vi "Main.vi"(8 "error in":errorcluster, 11 "TopUI in":refnum<class "TopUI.lvclass">) -> (0 "error out":errorcluster, 3 "TopUI out":refnum<class "TopUI.lvclass">)   [LabVIEW 2019, in "TopUI.lvclass"]
doc: "The <b>Queued Message Handler</b> of the Worker that owns this VI."
uses:
  TopUI.lvclass
  C:/Program Files (x86)/National Instruments/LabVIEW 2019/vi.lib/addons/_Workers/Library/Classes/Worker/Worker.lvclass
  Initialization Data.ctl
  Response Cases.ctl
  rql_AC_Init.ctl
  TopUI.lvclass/TopUI.ctl
  rql_PM_Init.ctl
  rql_Load_Init.ctl
  rql_Rly_Init.ctl
  rql_CK_Type.ctl
  rql_AC_Preset.ctl
  rql_AC_Setup.ctl
  rql_PM_Voltage.ctl
  rql_PM_Current.ctl
  rql_PM_Power.ctl
  rql_PM_P.F.ctl
  rql_PM_Integrate.ctl
  rql_Load_Preset.ctl
  rql_Source_Ctrl.ctl
  rql_Load_Ctrl.ctl
  edbbe92a-6b9d-4f6a-b93a-ee9e5c5b7043.vi
  a3d05794-377f-4d22-b0ed-f270b59c785d.vi
  cac2f185-9852-42f1-bdde-2e867e5f0e86.vi
  326cd913-60c8-4f39-b041-9c4d2d313c5b.vi
  79ea6008-7afc-4004-bcc9-20c1de84bee4.vi
  92421e1f-ff6e-4b36-ba89-2eae84818746.vi
  846e5152-3c31-460c-8b34-4e4e2cc733f6.vi
  63e7fb60-e3b3-40f1-8995-d086ce088de3.vi
  6951fa56-5880-407f-8b78-e7ddc2d94f99.vi
  e5f76952-d3c5-4b56-9ea4-0d04458dc5f7.vi
  <vilib>/Instr/_visa.llb/VISA Configure Serial Port (Instr).vi
  <instrlib>/Yokogawa WT300 Series/Public/Utility/Function/Create Function String (Voltage).vi
  <instrlib>/Yokogawa WT300 Series/Public/Data/Read Measurement (Normal).vi
  <instrlib>/Yokogawa WT300 Series/Public/Utility/Function/Create Function String (Current).vi
  <instrlib>/Yokogawa WT300 Series/Public/Utility/Function/Create Function String (Power).vi
  <instrlib>/Yokogawa WT300 Series/Public/Utility/Function/Create Function String (Integrate).vi
  <vilib>/addons/_Workers/Library/Classes/Message Queue/Message Queue.lvclass
  <instrlib>/Yokogawa WT300 Series/Yokogawa WT300 Series.lvlib
  <instrlib>/Prodigit 331xF Series/Prodigit 331xF Series.lvlib
  <vilib>/addons/_Workers/Debugger/Debug Client/Debug Client.lvlib
panel:
  in  "Load":u16(ring) items=["A,B,C", "D,E,F", "G,H,I"]
  in  "Source":u16(ring) items=["A,B,C", "D,E,F", "G,H,I"]
  in  "InputType":u16(ring) items=["115V,60Hz", "230V,50Hz", "115V,60Hz & 230V,50Hz"]
  in  "OutputType":enum32{"Standard", "TypeC"}(tab)
  in  "MaxLoad":dbl
  in  "Vo":dbl
  in  "Vo_Hi":dbl
  in  "MaxLoad C":dbl
  in  "Initialization Data":T1
  in  "Worker Alias":string="TopUI"
  in  "ST":bool
  in  "Rly":refnum<visa-resource-name>
  in  "Load":refnum<visa-resource-name>
  in  "PM":refnum<visa-resource-name>
  in  "AC":refnum<visa-resource-name>
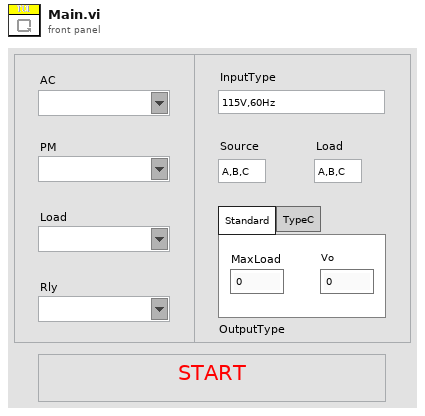
[diagram p1: front panel]
types:
  T1 = typedef "TopUI.lvclass/Initialization Data.ctl" = cluster{"Response Cases":T2}
  T2 = typedef "TopUI.lvclass/Response Cases.ctl" = cluster{"Placeholder - Can be deleted":string}
  T3 = typedef "TopUI.lvclass/rql_AC_Init.ctl" = cluster{"String":string}
  T4 = typedef "TopUI.lvclass/rql_PM_Init.ctl" = cluster{"String":string}
  T5 = typedef "TopUI.lvclass/rql_Load_Init.ctl" = cluster{"String":string}
  T6 = typedef "TopUI.lvclass/rql_Rly_Init.ctl" = cluster{"String":string}
  T7 = typedef "TopUI.lvclass/rql_CK_Type.ctl" = cluster{"String":string}
  T8 = typedef "TopUI.lvclass/rql_AC_Preset.ctl" = cluster{"String":string}
  T9 = enum16{":SOUR:RANG LOW;", ":SOUR:RANG HIGH;", ":SOUR:RANG AUTO;"}
  T10 = typedef "TopUI.lvclass/rql_AC_Setup.ctl" = cluster{"String":string}
  T11 = enum16{"SetRange", "SetVoltage", "SetFreq", "OUTP", "TurnOn"}
  T12 = typedef "TopUI.lvclass/rql_PM_Voltage.ctl" = cluster{"String":string}
  T13 = typedef "TopUI.lvclass/rql_PM_Current.ctl" = cluster{"String":string}
  T14 = typedef "TopUI.lvclass/rql_PM_Power.ctl" = cluster{"String":string}
  T15 = typedef "TopUI.lvclass/rql_PM_P.F.ctl" = cluster{"String":string}
  T16 = typedef "TopUI.lvclass/rql_PM_Integrate.ctl" = cluster{"String":string}
  T17 = typedef "TopUI.lvclass/rql_Load_Preset.ctl" = cluster{"String":string}
  T18 = typedef "TopUI.lvclass/rql_Source_Ctrl.ctl" = cluster{"String":string}
  T19 = typedef "TopUI.lvclass/rql_Load_Ctrl.ctl" = cluster{"String":string}
  T20 = cluster{"RangSelect":enum16{":SOUR:RANG LOW;", ":SOUR:RANG HIGH;", ":SOUR:RANG AUTO;"}, "Volt(V)":string, "Freq(Hz)":string, "OutpSlect":enum16{":SOUR:TURN OFF;", ":SOUR:TURN ON;"}, "TurnSlect":enum16{":SOUR:TURN OFF;", ":SOUR:TURN ON;"}}
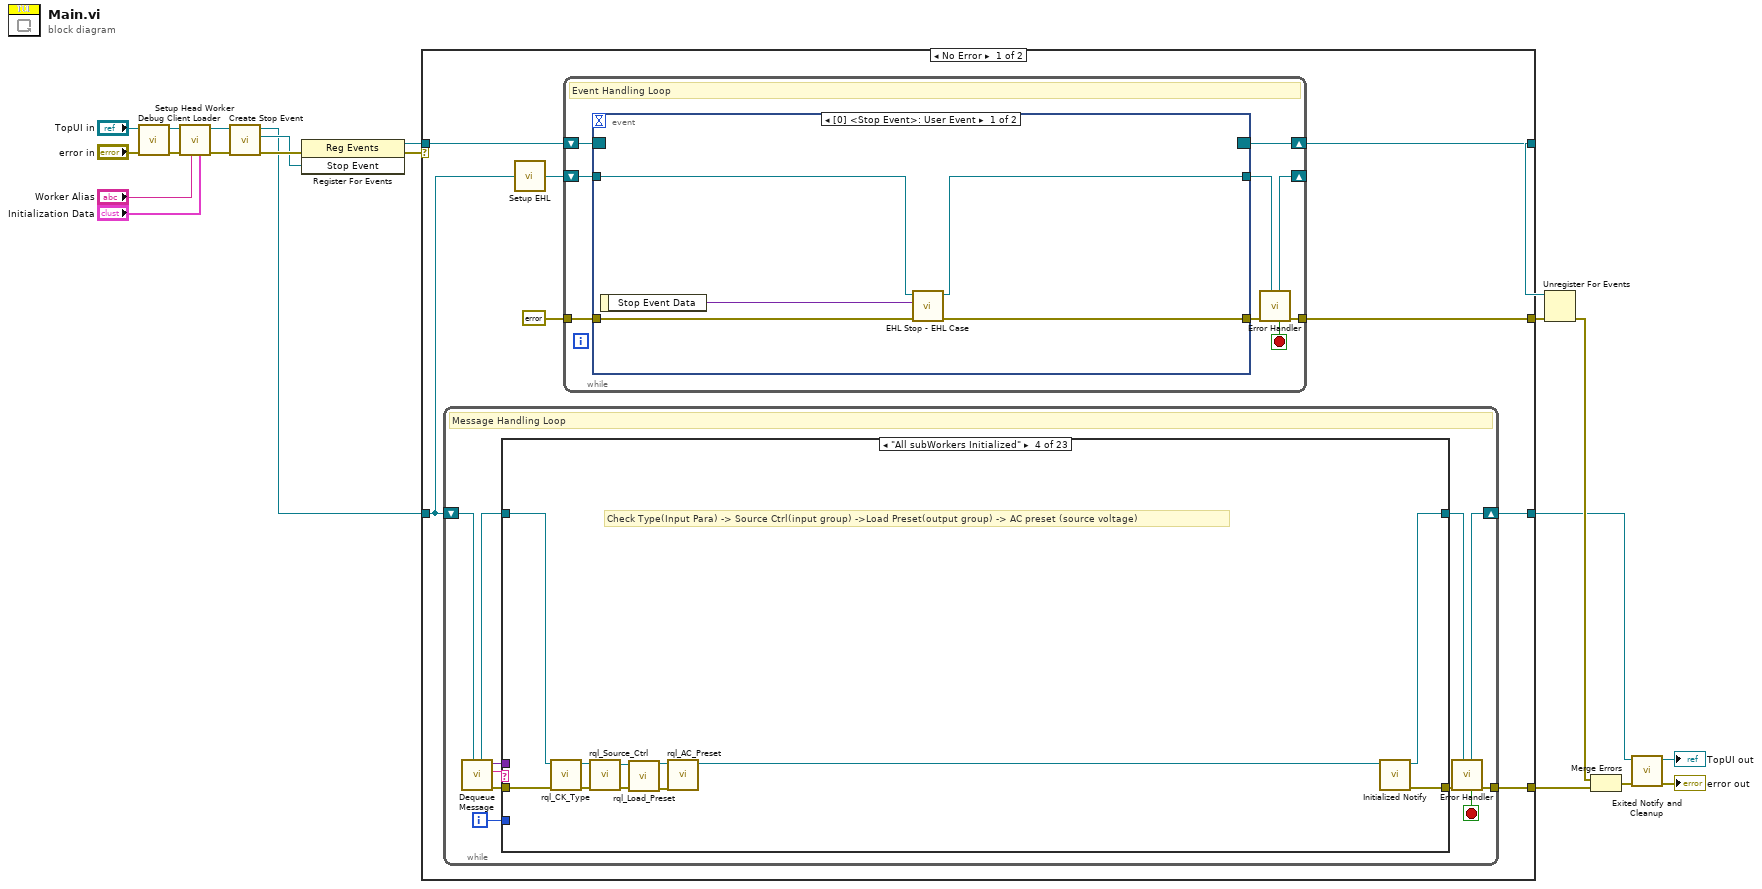
[diagram p0: block diagram]
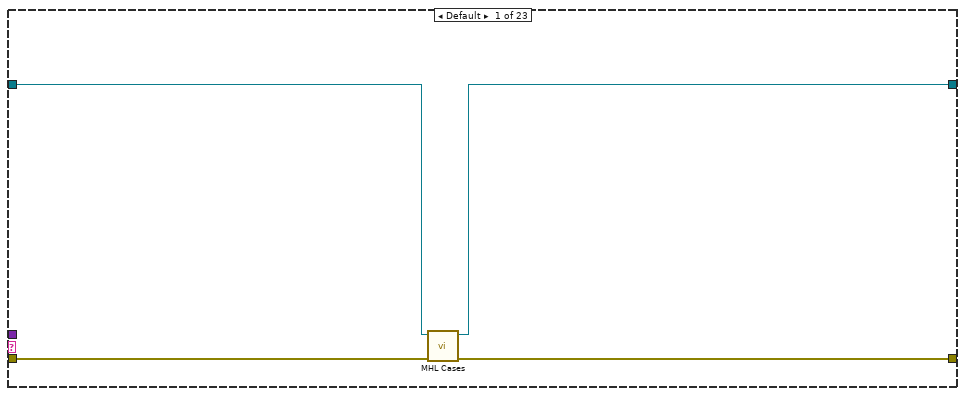
[diagram p2: hidden frame]
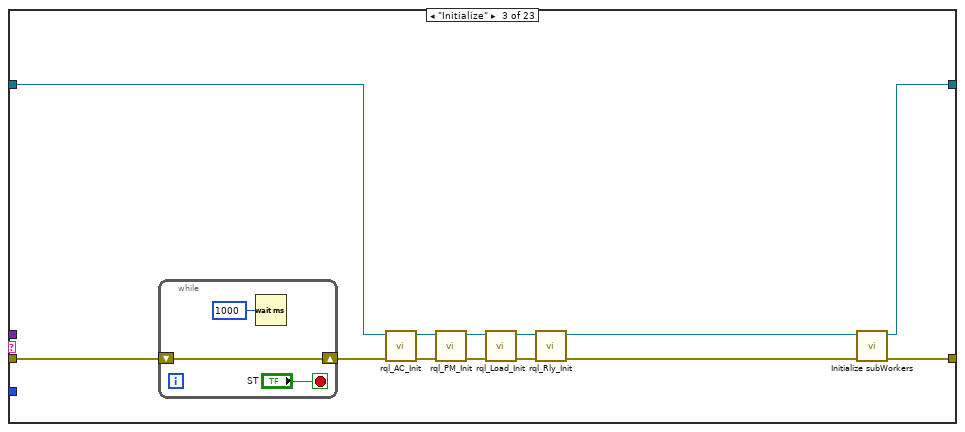
[diagram p4: hidden frame]
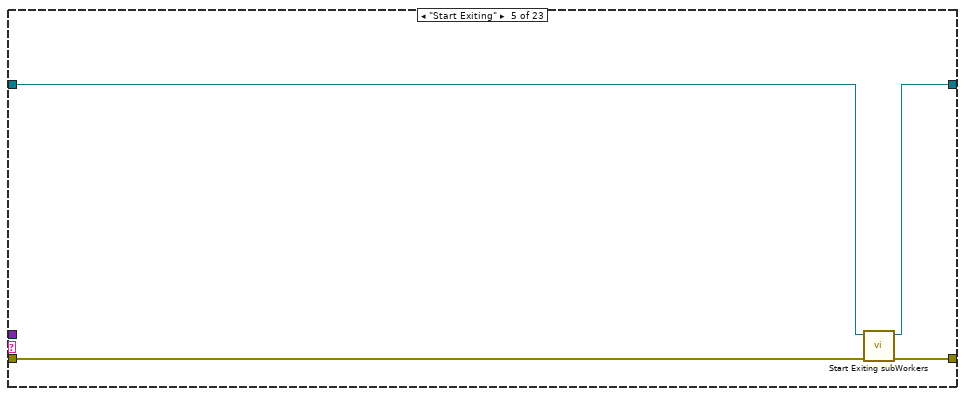
[diagram p5: hidden frame]
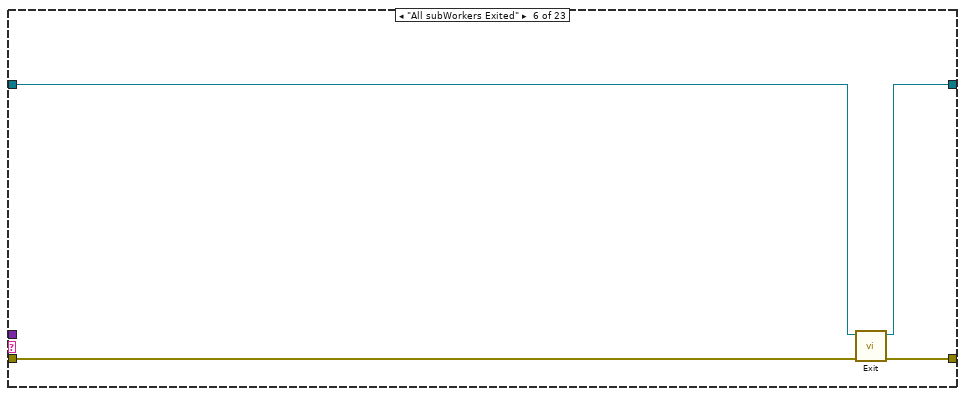
[diagram p6: hidden frame]
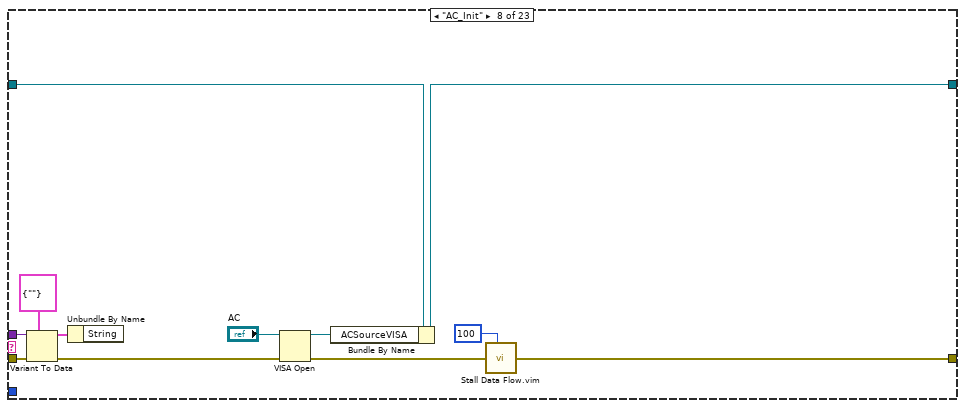
[diagram p8: hidden frame]
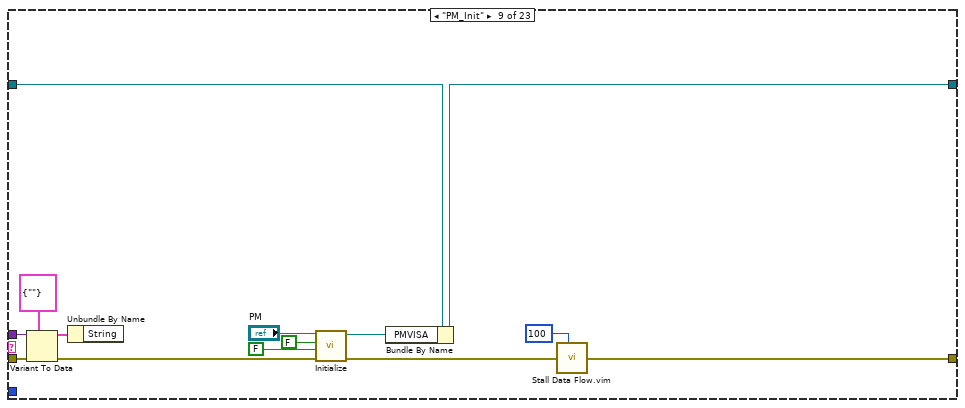
[diagram p9: hidden frame]
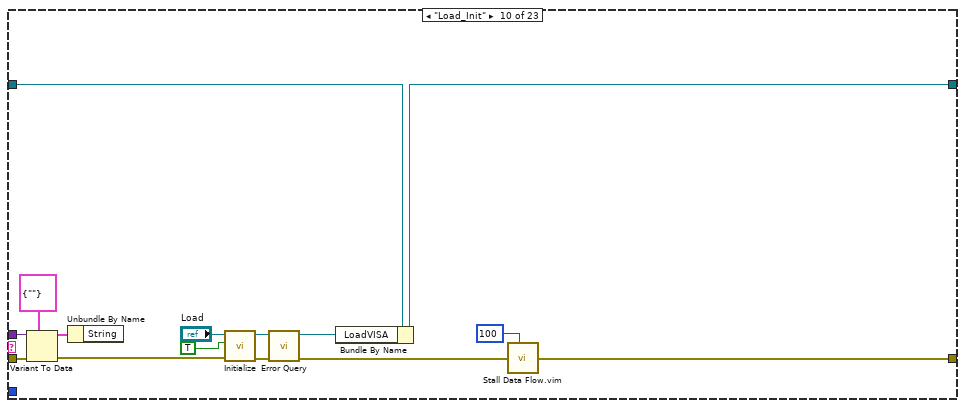
[diagram p10: hidden frame]
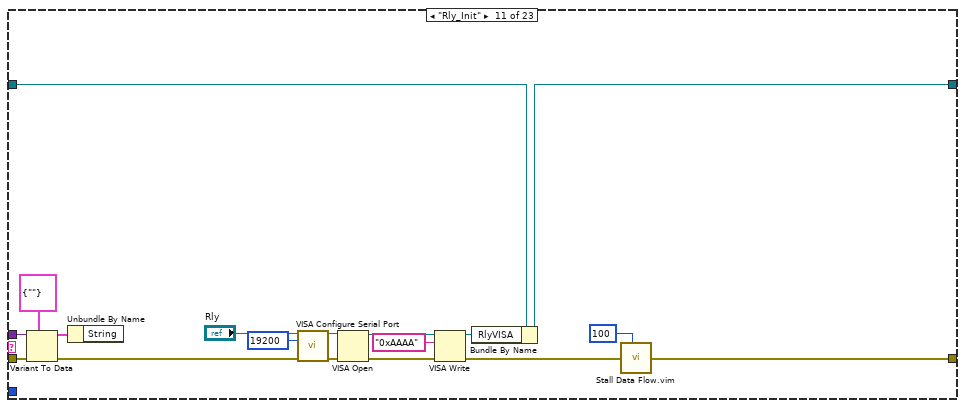
[diagram p11: hidden frame]
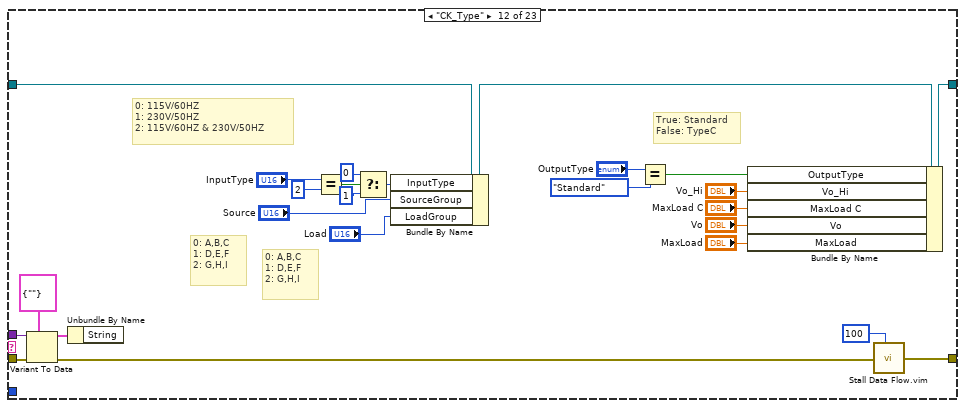
[diagram p12: hidden frame]
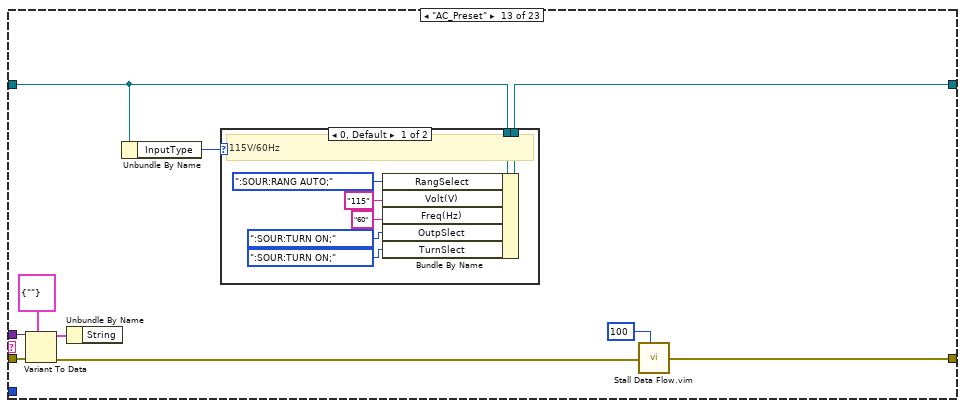
[diagram p13: hidden frame]
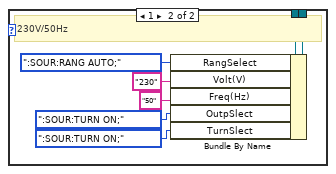
[diagram p14: hidden frame]
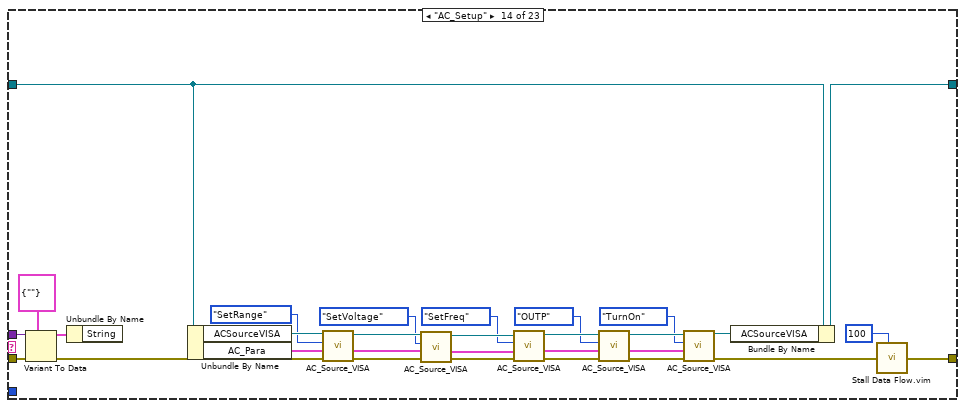
[diagram p15: hidden frame]
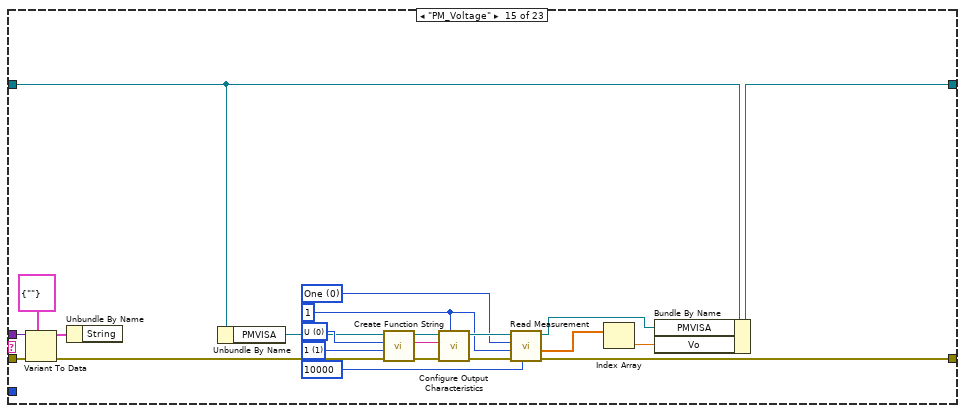
[diagram p16: hidden frame]
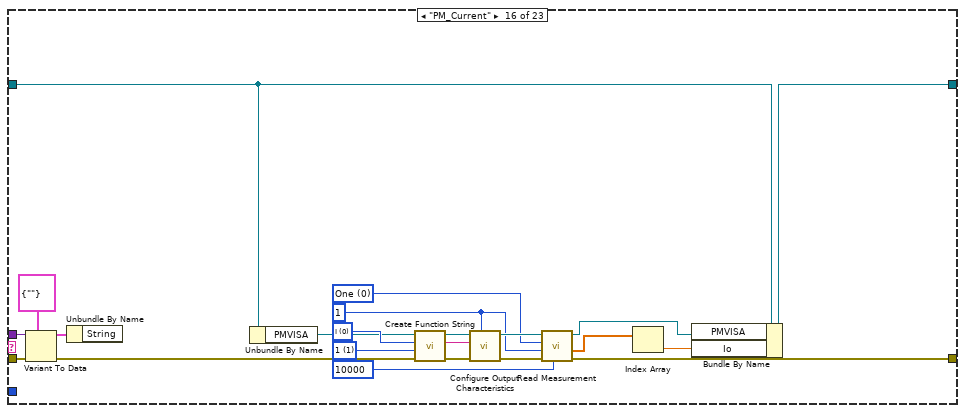
[diagram p17: hidden frame]
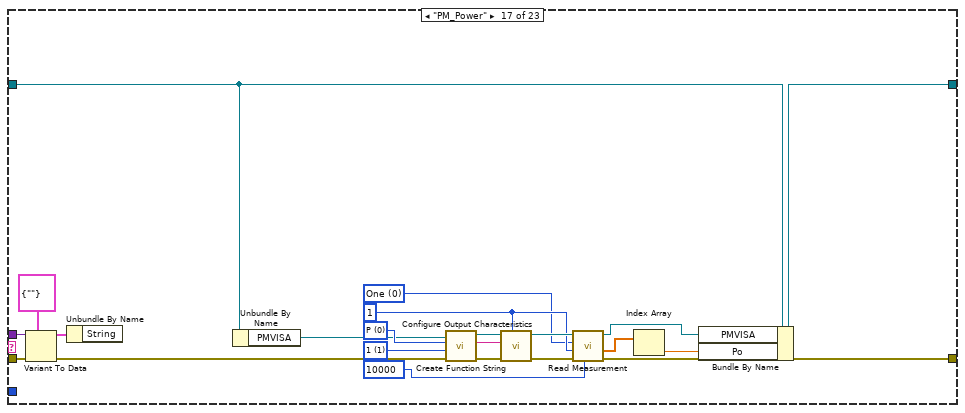
[diagram p18: hidden frame]
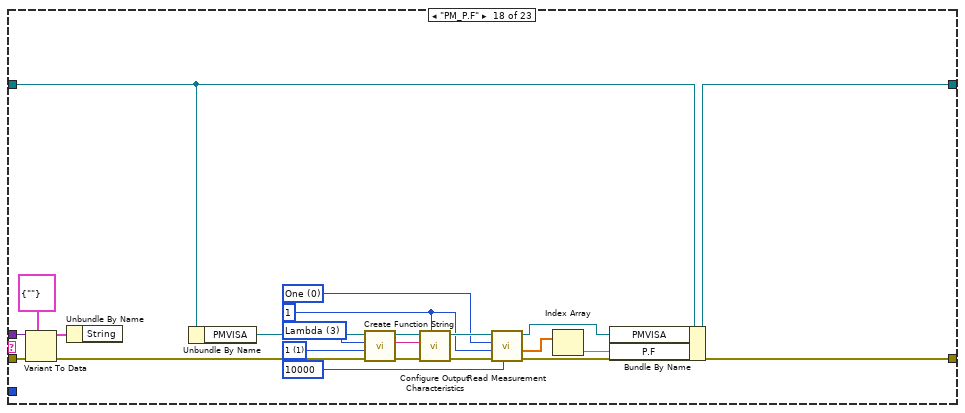
[diagram p19: hidden frame]
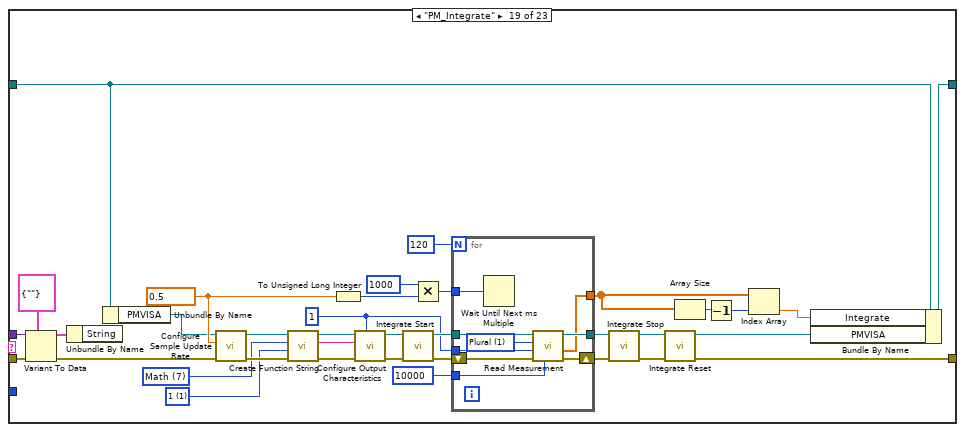
[diagram p20: hidden frame]
diagram:
  n1 = call <vilib>:"Debug Client Loader.vi"("error in (no error)"="error in", "Worker_"="TopUI in") -> ("error out"=w8:errorcluster, "Worker_out"=w7:refnum<class "TopUI.lvclass">)  [unwired: 8 in]
  n2 = call-dynamic "Setup Head Worker.vi"("Initalization Data"="Initialization Data", "Worker Alias"="Worker Alias", "error in"=w8, "Worker_"=w7) -> ("error out"=w3:errorcluster, "Worker_out"=w4:refnum<class "TopUI.lvclass">)  [unwired: 6 in]
  n3 = call-dynamic "Create Stop Event.vi"("error in"=w3, "Worker"=w4) -> ("error out"=w16:errorcluster, "Stop Event"=w13:refnum<user-event>, "Worker out"=w10:refnum<class "TopUI.lvclass">)  [unwired: 7 in]
  n4 = register-events(error in=w16, w13) -> (reference out=w15:refnum<event-registration>, error out=w9:errorcluster)  [unwired: 1 in]
  n5 = case shown="No Error" w9 {
    tunnel: w10 -> [w24 w447]
    tunnel: [w22 w448] -> w14
    tunnel: w15 -> [w29 w449]
    tunnel: [w26 w450] -> w20
    tunnel: [w28 w449] -> w19
    tunnel: [w23 w446] -> w17
    selector: w9 -> [_ w450]
    frame No Error {
      n6 = while {
        shift-right: [w38] -> w23
        shift-left: w24 -> [w40]
        tunnel: [w39] -> w22
        i -> [w31]
        stop <- w32 stop-if-true
        # "Message Handling Loop"
        n7 = call-dynamic "Dequeue Message.vi"("Worker"=w40) -> ("error out"=w37:errorcluster, "Case out"=w33:string, "Data out"=w30:variant, "Worker out"=w35:refnum<class "TopUI.lvclass">)  [unwired: 6 in, 1 out]
        n8 = case "Worker MHL Case Structure (DO NOT CHANGE LABEL NAME)" shown="\"All subWorkers Initialized\"" w33 {
          tunnel: w37 -> [w44 w45 w47 w71 w74 w81 w83 w87 w99 w113 w128 w146 w171 w195 w225 w247 w269 w291 w313 w369 w408 w422 w424]
          tunnel: [w41 w45 w59 w73 w77 w80 w83 w89 w108 w123 w137 w166 w176 w220 w233 w255 w276 w298 w319 w363 w403 w412 w424] -> w36
          tunnel: w35 -> [w43 w46 w49 w70 w75 w79 w82 w92 w104 w117 w136 w159 w174 w199 w230 w252 w274 w296 w324 w362 w402 w410 w423]
          tunnel: [w42 w46 w56 w72 w76 w78 w82 w90 w103 w115 w135 w160 w173 w197 w227 w249 w273 w295 w323 w360 w401 w409 w423] -> w34
          tunnel: w31 -> [_ _ _ _ _ _ _ _ _ _ _ _ _ _ _ _ _ _ _ _ _ _ _]
          tunnel: w30 -> [_ _ _ _ _ _ _ w85 w97 w111 w126 w143 w168 w193 w223 w244 w267 w289 w311 w367 w406 w420 _]
          frame Default {
            # "Base Class MHL Cases\nContains the MHL Cases of this Worker's base class."
            n9 = call-dynamic "MHL Cases.vi"("error in"=w44, "Worker in"=w43) -> ("error out"=w41:errorcluster, "Worker out"=w42:refnum<class "TopUI.lvclass">)  [unwired: 8 in]
          }
          frame "------------ FRAMEWORK CASES -----------" {
            # "Start of Workers Framework Cases"
          }
          frame "Initialize" {
            # "The first user case called when this Worker is loaded.\nThe end of this case (or series of cases) should call 'Initialize subWorkers.vi'"
            n10 = while {
              shift-right: [w62] -> w48
              shift-left: w47 -> [w62]
              stop <- "ST" stop-if-true
              n11 = Wait (ms)(milliseconds to wait=u32 1000) -> ()  [unwired: 1 out]
            }
            n12 = call "rql_AC_Init.vi"("error in"=w48, "TopUI in"=w49) -> ("error out"=w58:errorcluster, "dup TopUI out"=w57:refnum<class "TopUI.lvclass">)  [unwired: 8 in]
            n13 = call "rql_PM_Init.vi"("error in"=w58, "TopUI in"=w57) -> ("error out"=w55:errorcluster, "dup TopUI out"=w54:refnum<class "TopUI.lvclass">)  [unwired: 8 in]
            n14 = call "rql_Load_Init.vi"("error in"=w55, "TopUI in"=w54) -> ("error out"=w53:errorcluster, "dup TopUI out"=w52:refnum<class "TopUI.lvclass">)  [unwired: 8 in]
            n15 = call "rql_Rly_Init.vi"("error in"=w53, "TopUI in"=w52) -> ("error out"=w50:errorcluster, "dup TopUI out"=w51:refnum<class "TopUI.lvclass">)  [unwired: 8 in]
            n16 = call-dynamic "Initialize subWorkers.vi"("error in"=w50, "Worker"=w51) -> ("error out"=w59:errorcluster, "dup Worker out"=w56:refnum<class "TopUI.lvclass">)  [unwired: 8 in]
          }
          frame "All subWorkers Initialized" {
            # "Check Type(Input Para) -> Source Ctrl(input group) ->Load Preset(output group) -> AC preset (source voltage)"
            # "All of this Worker's statically-linked subWorkers have been successfully initialized.\nThis case should now call 'Initialized Notify.vi'"
            n17 = call "rql_CK_Type.vi"("error in"=w71, "TopUI in"=w70) -> ("error out"=w69:errorcluster, "dup TopUI out"=w68:refnum<class "TopUI.lvclass">)  [unwired: 8 in]
            n18 = call "rql_Source_Ctrl.vi"("error in"=w69, "TopUI in"=w68) -> ("error out"=w65:errorcluster, "dup TopUI out"=w66:refnum<class "TopUI.lvclass">)  [unwired: 8 in]
            n19 = call "rql_Load_Preset.vi"("error in"=w65, "TopUI in"=w66) -> ("error out"=w64:errorcluster, "dup TopUI out"=w63:refnum<class "TopUI.lvclass">)  [unwired: 8 in]
            n20 = call "rql_AC_Preset.vi"("error in"=w64, "TopUI in"=w63) -> ("dup TopUI out"=w67:refnum<class "TopUI.lvclass">)  [unwired: 8 in, 1 out]
            n21 = call-dynamic "Initialized Notify.vi"("Worker"=w67) -> ("error out"=w73:errorcluster, "dup Worker out"=w72:refnum<class "TopUI.lvclass">)  [unwired: 9 in]
          }
          frame "Start Exiting" {
            # "This Worker has been requested to exit. \nThe end of this case (or series of cases) should call 'Start Exiting subWorkers.vi'"
            n22 = call-dynamic "Start Exiting subWorkers.vi"("error_in"=w74, "Worker"=w75) -> ("error out"=w77:errorcluster, "dup Worker out"=w76:refnum<class "TopUI.lvclass">)  [unwired: 8 in]
          }
          frame "All subWorkers Exited" {
            # "All of this Worker's subWorkers have successfully exited. \nThe end of this case (or series of cases) should call 'Exit.vi'"
            n23 = call-dynamic "Exit.vi"("error_in"=w81, "Worker"=w79) -> ("error out"=w80:errorcluster, "dup Worker out"=w78:refnum<class "TopUI.lvclass">)  [unwired: 8 in]
          }
          frame "------------- LOCAL API CASES -------------" {
            # "Start of Workers Local API Cases"
          }
          frame "AC_Init" {
            # "Workers Local API Request Case"
            n24 = Variant To Data(error in=w87, type=T3 {"String"=""} ("Data"), Variant=w85) -> (data=w88:T3, error out=w86:errorcluster)
            n25 = Unbundle By Name(w88) -> ()  [unwired: 1 out]
            n26 = VISA Open(error in (no error)=w86, VISA resource name="AC") -> (VISA resource name=w91:refnum<visa-resource-name>, error out=w94:errorcluster)  [unwired: 3 in]
            n27 = Bundle By Name(cluster=w92, "ACSourceVISA"=w91) -> (w90:refnum<class "TopUI.lvclass">)
            n28 = call "Stall Data Flow.vim"("value in"=w94, "milliseconds to wait"=u32 100) -> ("value out"=w89:errorcluster)  [unwired: 1 out]
          }
          frame "PM_Init" {
            # "Workers Local API Request Case"
            n29 = Variant To Data(error in=w99, type=T4 {"String"=""} ("Data"), Variant=w97) -> (data=w100:T4, error out=w96:errorcluster)
            n30 = Unbundle By Name(w100) -> ()  [unwired: 1 out]
            n31 = call <instrlib>:"Initialize.vi"("error in (no error)"=w96, "Reset (True)"=FALSE, "ID Query (True)"=FALSE, "VISA resource name"="PM") -> ("error out"=w105:errorcluster, "VISA resource name out"=w102:refnum<visa-resource-name>)  [unwired: 6 in]
            n32 = Bundle By Name(cluster=w104, "PMVISA"=w102) -> (w103:refnum<class "TopUI.lvclass">)
            n33 = call "Stall Data Flow.vim"("value in"=w105, "milliseconds to wait"=u32 100) -> ("value out"=w108:errorcluster)  [unwired: 1 out]
          }
          frame "Load_Init" {
            # "Workers Local API Request Case"
            n34 = Variant To Data(error in=w113, type=T5 {"String"=""} ("Data"), Variant=w111) -> (data=w114:T5, error out=w112:errorcluster)
            n35 = Unbundle By Name(w114) -> ()  [unwired: 1 out]
            n36 = call <instrlib>:"Initialize.vi"("error in (no error)"=w112, "ID Query (True)"=TRUE, "VISA resource name"="Load") -> ("error out"=w119:errorcluster, "VISA resource name out"=w122:refnum<visa-resource-name>)  [unwired: 7 in]
            n37 = call <instrlib>:"Error Query.vi"("error in (no error)"=w119, "VISA resource name"=w122) -> ("error out"=w118:errorcluster, "VISA resource name out"=w116:refnum<visa-resource-name>)  [unwired: 6 in, 2 out]
            n38 = Bundle By Name(cluster=w117, "LoadVISA"=w116) -> (w115:refnum<class "TopUI.lvclass">)
            n39 = call "Stall Data Flow.vim"("value in"=w118, "milliseconds to wait"=u32 100) -> ("value out"=w123:errorcluster)  [unwired: 1 out]
          }
          frame "Rly_Init" {
            # "Workers Local API Request Case"
            n40 = Variant To Data(error in=w128, type=T6 {"String"=""} ("Data"), Variant=w126) -> (data=w129:T6, error out=w127:errorcluster)
            n41 = Unbundle By Name(w129) -> ()  [unwired: 1 out]
            n42 = call-poly "VISA Configure Serial Port"("VISA resource name"="Rly", "baud rate (9600)"=u32 19200, "error in (no error)"=w127) -> ("VISA resource name out"=w141:refnum<visa-resource-name>, "error out"=w142:errorcluster)  [unwired: 6 in, 5 out]
            n43 = VISA Open(error in (no error)=w142, VISA resource name=w141) -> (VISA resource name=w131:refnum<visa-resource-name>, error out=w134:errorcluster)  [unwired: 3 in]
            n44 = VISA Write(VISA resource name=w131, write buffer="0xAAAA", error in (no error)=w134) -> (VISA resource name out=w132:refnum<visa-resource-name>, error out=w133:errorcluster)  [unwired: 1 out]
            n45 = Bundle By Name(cluster=w136, "RlyVISA"=w132) -> (w135:refnum<class "TopUI.lvclass">)
            n46 = call "Stall Data Flow.vim"("value in"=w133, "milliseconds to wait"=u32 100) -> ("value out"=w137:errorcluster)  [unwired: 1 out]
          }
          frame "CK_Type" {
            # "0: A,B,C\n1: D,E,F\n2: G,H,I"
            # "0: A,B,C\n1: D,E,F\n2: G,H,I"
            # "True: Standard\nFalse: TypeC"
            # "0: 115V/60HZ\n1: 230V/50HZ\n2: 115V/60HZ & 230V/50HZ"
            # "Workers Local API Request Case"
            n47 = Variant To Data(error in=w146, type=T7 {"String"=""} ("Data"), Variant=w143) -> (data=w147:T7, error out=w145:errorcluster)
            n48 = Unbundle By Name(w147) -> ()  [unwired: 1 out]
            n49 = Equal?(x="InputType", y=u16 2) -> (x = y?=w155:bool)
            n50 = Select(t=u16 0 ("y"), s=w155, f=u16 1 ("y")) -> (s? t:f=w152:u16)
            n51 = Bundle By Name(cluster=w159, "InputType"=w152, "SourceGroup"="Source", "LoadGroup"="Load") -> (w158:refnum<class "TopUI.lvclass">)
            n52 = Equal?(x="OutputType", y=enum32{"Standard", "TypeC"}."Standard") -> (x = y?=w165:bool)
            n53 = Bundle By Name(cluster=w158, "OutputType"=w165, "Vo_Hi"="Vo_Hi", "MaxLoad C"="MaxLoad C", "Vo"="Vo", "MaxLoad"="MaxLoad") -> (w160:refnum<class "TopUI.lvclass">)
            n54 = call "Stall Data Flow.vim"("value in"=w145, "milliseconds to wait"=u32 100) -> ("value out"=w166:errorcluster)  [unwired: 1 out]
          }
          frame "AC_Preset" {
            # "Workers Local API Request Case"
            n55 = Variant To Data(error in=w171, type=T8 {"String"=""} ("Data"), Variant=w168) -> (data=w172:T8, error out=w170:errorcluster)
            n56 = Unbundle By Name(w172) -> ()  [unwired: 1 out]
            n57 = Unbundle By Name(w174) -> ("InputType"=w175:u16)
            n58 = case shown="0, Default" w175 {
              tunnel: w174 -> [w184 w191]
              tunnel: [w183 w190] -> w173
              frame 0, Default {
                # "115V/60Hz"
                n59 = Bundle By Name(cluster=w184, "RangSelect"=T9.":SOUR:RANG AUTO;" ("AC_Para.RangSelect"), "Volt(V)"="115" ("AC_Para.Volt(V)"), "Freq(Hz)"="60" ("AC_Para.Freq(Hz)"), "OutpSlect"=enum16{":SOUR:TURN OFF;", ":SOUR:TURN ON;"}.":SOUR:TURN ON;" ("AC_Para.OutpSlect"), "TurnSlect"=enum16{":SOUR:TURN OFF;", ":SOUR:TURN ON;"}.":SOUR:TURN ON;" ("AC_Para.TurnSlect")) -> (w183:refnum<class "TopUI.lvclass">)
              }
              frame 1 {
                # "230V/50Hz"
                n60 = Bundle By Name(cluster=w191, "RangSelect"=T9.":SOUR:RANG AUTO;" ("AC_Para.RangSelect"), "Volt(V)"="230" ("AC_Para.Volt(V)"), "Freq(Hz)"="50" ("AC_Para.Freq(Hz)"), "OutpSlect"=enum16{":SOUR:TURN OFF;", ":SOUR:TURN ON;"}.":SOUR:TURN ON;" ("AC_Para.OutpSlect"), "TurnSlect"=enum16{":SOUR:TURN OFF;", ":SOUR:TURN ON;"}.":SOUR:TURN ON;" ("AC_Para.TurnSlect")) -> (w190:refnum<class "TopUI.lvclass">)
              }
            }
            n61 = call "Stall Data Flow.vim"("value in"=w170, "milliseconds to wait"=u32 100) -> ("value out"=w176:errorcluster)  [unwired: 1 out]
          }
          frame "AC_Setup" {
            # "Workers Local API Request Case"
            n62 = Variant To Data(error in=w195, type=T10 {"String"=""} ("Data"), Variant=w193) -> (data=w196:T10, error out=w194:errorcluster)
            n63 = Unbundle By Name(w196) -> ()  [unwired: 1 out]
            n64 = Unbundle By Name(w199) -> ("ACSourceVISA"=w219:refnum<visa-resource-name>, "AC_Para"=w218:T20)
            n65 = call "AC_Source_VISA.vi"("error_in"=w194, "Parameter"=w218, "Mode"=T11."SetRange", "VISA_in"=w219) -> ("error_out"=w216:errorcluster, "Parameter 2"=w208:T20, "VISA_out"=w215:refnum<visa-resource-name>)  [unwired: 1 in]
            n66 = call "AC_Source_VISA.vi"("error_in"=w216, "Parameter"=w208, "Mode"=T11."SetVoltage", "VISA_in"=w215) -> ("error_out"=w213:errorcluster, "Parameter 2"=w207:T20, "VISA_out"=w214:refnum<visa-resource-name>)  [unwired: 1 in]
            n67 = call "AC_Source_VISA.vi"("error_in"=w213, "Parameter"=w207, "Mode"=T11."SetFreq", "VISA_in"=w214) -> ("error_out"=w211:errorcluster, "Parameter 2"=w206:T20, "VISA_out"=w212:refnum<visa-resource-name>)  [unwired: 1 in]
            n68 = call "AC_Source_VISA.vi"("error_in"=w211, "Parameter"=w206, "Mode"=T11."OUTP", "VISA_in"=w212) -> ("error_out"=w209:errorcluster, "Parameter 2"=w205:T20, "VISA_out"=w210:refnum<visa-resource-name>)  [unwired: 1 in]
            n69 = call "AC_Source_VISA.vi"("error_in"=w209, "Parameter"=w205, "Mode"=T11."TurnOn", "VISA_in"=w210) -> ("error_out"=w204:errorcluster, "VISA_out"=w198:refnum<visa-resource-name>)  [unwired: 1 in, 1 out]
            n70 = Bundle By Name(cluster=w199, "ACSourceVISA"=w198) -> (w197:refnum<class "TopUI.lvclass">)
            n71 = call "Stall Data Flow.vim"("value in"=w204, "milliseconds to wait"=u32 100) -> ("value out"=w220:errorcluster)  [unwired: 1 out]
          }
          frame "PM_Voltage" {
            w235 = 1 items=["1"=1, "2"=2, "3"=3, "Sigma A"=4] ("Element (1: 1)")
            w234 = 0 items=["U", "UPPeak", "UMPeak"] ("Function (0: U)")
            w237 = 1 ("Item (1)")
            w236 = 0 items=["One", "Plural"] ("Measure Item")
            # "Workers Local API Request Case"
            n72 = Variant To Data(error in=w225, type=T12 {"String"=""} ("Data"), Variant=w223) -> (data=w226:T12, error out=w224:errorcluster)
            n73 = Unbundle By Name(w226) -> ()  [unwired: 1 out]
            n74 = Unbundle By Name(w230) -> ("PMVISA"=w232:refnum<visa-resource-name>)
            n75 = call-poly <instrlib>:"Create Function String.vi"("error in (no error)"=w224, "Element (1: 1)"=w235, "Function (0: U)"=w234, "VISA resource name"=w232) -> ("error out"=w242:errorcluster, "Function String"=w243:string, "VISA resource name out"=w241:refnum<visa-resource-name>)  [unwired: 5 in]
            n76 = call <instrlib>:"Configure Output Characteristics.vi"("Item (1)"=w237, "error in (no error)"=w242, "Function (Empty)"=w243, "VISA resource name"=w241) -> ("error out"=w240:errorcluster, "VISA resource name out"=w239:refnum<visa-resource-name>)  [unwired: 6 in]
            n77 = call-poly <instrlib>:"Read Measurement.vi"("Timeout (10000 ms)"=10000, "error in (no error)"=w240, "Number of Item (15)"=w237, "Measure Item (1: Plural)"=w236, "VISA resource name"=w239) -> ("error out"=w233:errorcluster, "Measurement"=w231:dbl[], "VISA resource name out"=w229:refnum<visa-resource-name>)  [unwired: 3 in, 1 out]
            n78 = Index Array(array=w231) -> (element=w228:dbl)  [unwired: 1 in]
            n79 = Bundle By Name(cluster=w230, "PMVISA"=w229, "Vo"=w228) -> (w227:refnum<class "TopUI.lvclass">)
          }
          frame "PM_Current" {
            w256 = 0 items=["I", "IPPeak", "IMPeak"] ("Function (0: I)")
            w257 = 1 items=["1"=1, "2"=2, "3"=3, "Sigma A"=4] ("Element (1: 1)")
            w259 = 1 ("Item (1)")
            w258 = 0 items=["One", "Plural"] ("Measure Item")
            # "Workers Local API Request Case"
            n80 = Variant To Data(error in=w247, type=T13 {"String"=""} ("Data"), Variant=w244) -> (data=w248:T13, error out=w246:errorcluster)
            n81 = Unbundle By Name(w248) -> ()  [unwired: 1 out]
            n82 = Unbundle By Name(w252) -> ("PMVISA"=w253:refnum<visa-resource-name>)
            n83 = call-poly <instrlib>:"Create Function String.vi"("error in (no error)"=w246, "Element (1: 1)"=w257, "Function (0: I)"=w256, "VISA resource name"=w253) -> ("error out"=w264:errorcluster, "Function String"=w265:string, "VISA resource name out"=w263:refnum<visa-resource-name>)  [unwired: 5 in]
            n84 = call <instrlib>:"Configure Output Characteristics.vi"("Item (1)"=w259, "error in (no error)"=w264, "Function (Empty)"=w265, "VISA resource name"=w263) -> ("error out"=w262:errorcluster, "VISA resource name out"=w261:refnum<visa-resource-name>)  [unwired: 6 in]
            n85 = call-poly <instrlib>:"Read Measurement.vi"("Timeout (10000 ms)"=10000, "error in (no error)"=w262, "Number of Item (15)"=w259, "Measure Item (1: Plural)"=w258, "VISA resource name"=w261) -> ("error out"=w255:errorcluster, "Measurement"=w254:dbl[], "VISA resource name out"=w251:refnum<visa-resource-name>)  [unwired: 3 in, 1 out]
            n86 = Index Array(array=w254) -> (element=w250:dbl)  [unwired: 1 in]
            n87 = Bundle By Name(cluster=w252, "PMVISA"=w251, "Io"=w250) -> (w249:refnum<class "TopUI.lvclass">)
          }
          frame "PM_Power" {
            w279 = 0 items=["P", "S", "Q", "Lambda", "Phi", "P+peak", "P-peak"] ("Function (0: P)")
            w280 = 1 items=["1"=1, "2"=2, "3"=3, "Sigma A"=4] ("Element (1: 1)")
            w281 = 1 ("Item (1)")
            w277 = 0 items=["One", "Plural"] ("Measure Item")
            # "Workers Local API Request Case"
            n88 = Variant To Data(error in=w269, type=T14 {"String"=""} ("Data"), Variant=w267) -> (data=w270:T14, error out=w268:errorcluster)
            n89 = Unbundle By Name(w270) -> ()  [unwired: 1 out]
            n90 = Unbundle By Name(w274) -> ("PMVISA"=w275:refnum<visa-resource-name>)
            n91 = call-poly <instrlib>:"Create Function String.vi"("error in (no error)"=w268, "Element (1: 1)"=w280, "Function (0: P)"=w279, "VISA resource name"=w275) -> ("error out"=w284:errorcluster, "Function String"=w283:string, "VISA resource name out"=w285:refnum<visa-resource-name>)  [unwired: 5 in]
            n92 = call <instrlib>:"Configure Output Characteristics.vi"("Item (1)"=w281, "error in (no error)"=w284, "Function (Empty)"=w283, "VISA resource name"=w285) -> ("error out"=w286:errorcluster, "VISA resource name out"=w287:refnum<visa-resource-name>)  [unwired: 6 in]
            n93 = call-poly <instrlib>:"Read Measurement.vi"("Timeout (10000 ms)"=10000, "error in (no error)"=w286, "Number of Item (15)"=w281, "Measure Item (1: Plural)"=w277, "VISA resource name"=w287) -> ("error out"=w276:errorcluster, "Measurement"=w282:dbl[], "VISA resource name out"=w271:refnum<visa-resource-name>)  [unwired: 3 in, 1 out]
            n94 = Index Array(array=w282) -> (element=w272:dbl)  [unwired: 1 in]
            n95 = Bundle By Name(cluster=w274, "PMVISA"=w271, "Po"=w272) -> (w273:refnum<class "TopUI.lvclass">)
          }
          frame "PM_P.F" {
            w299 = 3 items=["P", "S", "Q", "Lambda", "Phi", "P+peak", "P-peak"] ("Function (0: P)")
            w300 = 1 items=["1"=1, "2"=2, "3"=3, "Sigma A"=4] ("Element (1: 1)")
            w302 = 1 ("Item (1)")
            w301 = 0 items=["One", "Plural"] ("Measure Item")
            # "Workers Local API Request Case"
            n96 = Variant To Data(error in=w291, type=T15 {"String"=""} ("Data"), Variant=w289) -> (data=w292:T15, error out=w288:errorcluster)
            n97 = Unbundle By Name(w292) -> ()  [unwired: 1 out]
            n98 = Unbundle By Name(w296) -> ("PMVISA"=w297:refnum<visa-resource-name>)
            n99 = call-poly <instrlib>:"Create Function String.vi"("error in (no error)"=w288, "Element (1: 1)"=w300, "Function (0: P)"=w299, "VISA resource name"=w297) -> ("error out"=w307:errorcluster, "Function String"=w308:string, "VISA resource name out"=w306:refnum<visa-resource-name>)  [unwired: 5 in]
            n100 = call <instrlib>:"Configure Output Characteristics.vi"("Item (1)"=w302, "error in (no error)"=w307, "Function (Empty)"=w308, "VISA resource name"=w306) -> ("error out"=w305:errorcluster, "VISA resource name out"=w304:refnum<visa-resource-name>)  [unwired: 6 in]
            n101 = call-poly <instrlib>:"Read Measurement.vi"("Timeout (10000 ms)"=10000, "error in (no error)"=w305, "Number of Item (15)"=w302, "Measure Item (1: Plural)"=w301, "VISA resource name"=w304) -> ("error out"=w298:errorcluster, "Measurement"=w309:dbl[], "VISA resource name out"=w294:refnum<visa-resource-name>)  [unwired: 3 in, 1 out]
            n102 = Index Array(array=w309) -> (element=w293:dbl)  [unwired: 1 in]
            n103 = Bundle By Name(cluster=w296, "PMVISA"=w294, "P.F"=w293) -> (w295:refnum<class "TopUI.lvclass">)
          }
          frame "PM_Integrate" {
            w331 = 1 items=["1"=1, "2"=2, "3"=3, "Sigma A"=4] ("Element (1: 1)")
            w330 = 1 ("Item (1)")
            w332 = 7 items=["Time", "WP", "WP+", "WP-", "q", "q+", "q-", "Math"] ("Function (0: Time)")
            w338 = 0.5 items=["100m"=0.1, "250m"=0.25, "500m"=0.5, "1"=1.0, "2"=2.0, "5"=5.0] ("Update Rate (500m s)")
            # "Workers Local API Request Case"
            n104 = Variant To Data(error in=w313, type=T16 {"String"=""} ("Data"), Variant=w311) -> (data=w314:T16, error out=w312:errorcluster)
            n105 = Unbundle By Name(w314) -> ()  [unwired: 1 out]
            n106 = Unbundle By Name(w324) -> ("PMVISA"=w325:refnum<visa-resource-name>)
            n107 = call <instrlib>:"Configure Sample Update Rate.vi"("error in (no error)"=w312, "Update Rate (500m s)"=w338, "VISA resource name"=w325) -> ("error out"=w345:errorcluster, "VISA resource name out"=w344:refnum<visa-resource-name>)  [unwired: 7 in]
            n108 = call-poly <instrlib>:"Create Function String.vi"("error in (no error)"=w345, "Element (1: 1)"=w331, "Function (0: Time)"=w332, "VISA resource name"=w344) -> ("error out"=w333:errorcluster, "Function String"=w335:string, "VISA resource name out"=w334:refnum<visa-resource-name>)  [unwired: 5 in]
            n109 = To Unsigned Long Integer(number=w338) -> (unsigned 32bit integer=w329:u32)
            n110 = call <instrlib>:"Configure Output Characteristics.vi"("Item (1)"=w330, "error in (no error)"=w333, "Function (Empty)"=w335, "VISA resource name"=w334) -> ("error out"=w342:errorcluster, "VISA resource name out"=w343:refnum<visa-resource-name>)  [unwired: 6 in]
            n111 = call <instrlib>:"Integrate Start.vi"("error in (no error)"=w342, "VISA resource name"=w343) -> ("error out"=w341:errorcluster, "VISA resource name out"=w340:refnum<visa-resource-name>)  [unwired: 8 in]
            n112 = Multiply(x=u32 1000, y=w329) -> (x*y=w337:u32)
            n113 = for {
              N: 120 -> [_]
              tunnel: w340 -> [w352]
              tunnel: w330 -> [w351]
              tunnel: [w350] -> w318
              tunnel: w337 -> [w346]
              tunnel: 10000 ("Timeout (10000 ms)") -> [w348]
              tunnel: [w347] -> w326
              shift-right: [w349] -> w320
              shift-left: w341 -> [w354]
              w353 = 1 items=["One", "Plural"] ("Measure Item (1: Plural)")
              n114 = Wait Until Next ms Multiple(millisecond multiple=w346) -> ()  [unwired: 1 out]
              n115 = call-poly <instrlib>:"Read Measurement.vi"("Timeout (10000 ms)"=w348, "error in (no error)"=w354, "Number of Item (15)"=w351, "Measure Item (1: Plural)"=w353, "VISA resource name"=w352) -> ("error out"=w349:errorcluster, "Measurement"=w347:dbl[], "VISA resource name out"=w350:refnum<visa-resource-name>)  [unwired: 3 in, 1 out]
            }
            n116 = call <instrlib>:"Integrate Stop.vi"("error in (no error)"=w320, "VISA resource name"=w318) -> ("error out"=w321:errorcluster, "VISA resource name out"=w317:refnum<visa-resource-name>)  [unwired: 8 in]
            n117 = call <instrlib>:"Integrate Reset.vi"("error in (no error)"=w321, "VISA resource name"=w317) -> ("error out"=w319:errorcluster, "VISA resource name out"=w316:refnum<visa-resource-name>)  [unwired: 8 in]
            n118 = Array Size(array=w326) -> (size(s)=w328:i32)
            n119 = Decrement(x=w328) -> (x-1=w327:i32)
            n120 = Index Array(array=w326, index=w327) -> (element=w315:dbl)
            n121 = Bundle By Name(cluster=w324, "Integrate"=w315, "PMVISA"=w316) -> (w323:refnum<class "TopUI.lvclass">)
          }
          frame "Load_Preset" {
            # "Workers Local API Request Case"
            n122 = Variant To Data(error in=w369, type=T17 {"String"=""} ("Data"), Variant=w367) -> (data=w366:T17, error out=w357:errorcluster)
            n123 = Unbundle By Name(w362) -> ("VLoad"=w364:dbl, "LoadVISA"=w365:refnum<visa-resource-name>, "LoadGroup"=w358:u16)
            n124 = Unbundle By Name(w366) -> ()  [unwired: 1 out]
            n125 = case shown="0, Default" w358 {
              tunnel: w357 -> [w371 w373 w375]
              tunnel: [w371 w373 w375] -> w356
              tunnel: [1 ("x") 4 ("x") 7 ("x")] -> w355
              frame 0, Default {
              }
              frame 1 {
              }
              frame 2 {
              }
            }
            n126 = for {
              N: 3 -> [_]
              tunnel: w364 -> [w386]
              shift-right: [w379] -> w363
              shift-left: w356 -> [w394]
              tunnel: w365 -> [w393]
              tunnel: [w382] -> w361
              tunnel: w355 -> [w376]
              i -> [w378]
              w389 = u16 0 items=["Low", "High"] ("Current Level (F:Low)")
              w392 = 0 items=["Current", "Resistance", "Voltage", "Power"] ("Regulation Mode (0:Current)")
              n127 = Add(x=w376, y=w378) -> (x+y=w377:i32)
              n128 = call <instrlib>:"Configure Channel.vi"("error in (no error)"=w394, "Channel (0:Channel 1)"=w377, "VISA resource name"=w393) -> ("error out"=w391:errorcluster, "VISA resource name out"=w390:refnum<visa-resource-name>)  [unwired: 7 in]
              n129 = call <instrlib>:"Configure Operating Mode.vi"("error in (no error)"=w391, "Regulation Mode (0:Current)"=w392, "VISA resource name"=w390) -> ("error out"=w387:errorcluster, "VISA resource name out"=w388:refnum<visa-resource-name>)  [unwired: 7 in]
              n130 = call <instrlib>:"Configure Current.vi"("error in (no error)"=w387, "Current (0.0 A)"=w386, "Current Level (F:Low)"=w389, "VISA resource name"=w388) -> ("error out"=w383:errorcluster, "VISA resource name out"=w384:refnum<visa-resource-name>)  [unwired: 6 in]
              n131 = call <instrlib>:"Utility Load Switch.vi"("error in (no error)"=w383, "Load (F:Off)"=TRUE, "VISA resource name"=w384) -> ("error out"=w380:errorcluster, "VISA resource name out"=w382:refnum<visa-resource-name>)  [unwired: 7 in]
              n132 = call "Stall Data Flow.vim"("value in"=w380, "milliseconds to wait"=u32 100) -> ("value out"=w379:errorcluster)  [unwired: 1 out]
            }
            n133 = Bundle By Name(cluster=w362, "LoadVISA"=w361) -> (w360:refnum<class "TopUI.lvclass">)
          }
          frame "Source_Ctrl" {
            # "Source On"
            # "Workers Local API Request Case"
            n134 = Variant To Data(error in=w408, type=T18 {"String"=""} ("Data"), Variant=w406) -> (data=w405:T18, error out=w396:errorcluster)
            n135 = Unbundle By Name(w405) -> ()  [unwired: 1 out]
            n136 = Unbundle By Name(w402) -> ("RlyVISA"=w399:refnum<visa-resource-name>, "SourceGroup"=w397:u16)
            n137 = call "Source_Ctrl.vi"("Error in"=w396, "SourceGroup"=w397, "ON/OFF"=TRUE, "VISA in"=w399) -> ("error out"=w395:errorcluster, "VISA out"=w400:refnum<visa-resource-name>)  [unwired: 2 in]
            n138 = Bundle By Name(cluster=w402, "RlyVISA"=w400) -> (w401:refnum<class "TopUI.lvclass">)
            n139 = call "Stall Data Flow.vim"("value in"=w395, "milliseconds to wait"=u32 100) -> ("value out"=w403:errorcluster)  [unwired: 1 out]
          }
          frame "Load_Ctrl" {
            # "Workers Local API Request Case"
            n140 = Variant To Data(error in=w422, type=T19 {"String"=""} ("Data"), Variant=w420) -> (data=w419:T19, error out=w418:errorcluster)
            n141 = Unbundle By Name(w419) -> ()  [unwired: 1 out]
            n142 = Unbundle By Name(w410) -> ("LoadVISA"=w417:refnum<visa-resource-name>, "LoadGroup"=w415:u16)
            n143 = call "Load_Ctrl.vi"("Error in"=w418, "LoadGroup"=w415, "ON/OFF"=TRUE, "VISA in"=w417) -> ("error out"=w413:errorcluster, "VISA out"=w411:refnum<visa-resource-name>)  [unwired: 2 in]
            n144 = Bundle By Name(cluster=w410, "LoadVISA"=w411) -> (w409:refnum<class "TopUI.lvclass">)
            n145 = call "Stall Data Flow.vim"("value in"=w413, "milliseconds to wait"=u32 100) -> ("value out"=w412:errorcluster)  [unwired: 1 out]
          }
          frame "------------- RESPONSE CASES --------------" {
            # "Start of Workers Response Cases"
          }
        }
        n146 = call-dynamic "Error Handler.vi"("Worker"=w34, "error_in"=w36) -> ("error out"=w39:errorcluster, "Stop Loop"=w32:bool, "Worker out"=w38:refnum<class "TopUI.lvclass">)  [unwired: 7 in]
      }
      n147 = call-dynamic "Setup EHL.vi"("Worker"=w24) -> ("Worker out"=w25:refnum<class "TopUI.lvclass">)  [unwired: 14 in]
      n148 = while "Event Handling Loop" {
        shift-right: [w433] -> w28
        shift-left: w29 -> [w432]
        tunnel: [w428] -> w26
        tunnel: errorcluster {"status"=FALSE, "code"=0, "source"=""} ("error constant") -> [w430]
        shift-right: [w426] -> _
        shift-left: w25 -> [w431]
        stop <- w425 stop-if-true
        # "Event Handling Loop"
        n149 = event shown="[0] <Stop Event>: User Event" {
          selector: w432 -> [_ _]
          dyn-events: [_ _] -> w433
          timeout: _ -> [_ _]
          tunnel: [w437 w444] -> w429
          tunnel: w430 -> [w438 w443]
          tunnel: w431 -> [w436 w442]
          tunnel: [w435 w441] -> w427
          event User Event {
            # "EHL Stop Event. This EHL exits from this case."
            n150 = event-data() -> ("Stop Event Data"=w434:variant)  [unwired: 1 in]
            n151 = call-dynamic "EHL Stop - EHL Case.vi"("error in"=w438, "Stop Event Data"=w434, "Worker"=w436) -> ("error out"=w437:errorcluster, "Worker out"=w435:refnum<class "TopUI.lvclass">)  [unwired: 7 in]
          }
          event Panel Close? {
            # "Calls the Start Exiting case of this Worker. This will start the exiting sequence of this Worker."
            n152 = event-data() -> ()  [unwired: 1 in, 1 out]
            n153 = property class="TopUI"(reference=w442) -> (reference out=w440:refnum<class "TopUI.lvclass">, "Accessors:Read:Public API:Queue"=w439:refnum<class "Message Queue.lvclass">)  [unwired: 1 in, 1 out]
            n154 = call-dynamic "Worker Start Exiting.vi"("error_in"=w443, "Message Queue"=w439, "Worker"=w440) -> ("error out"=w444:errorcluster, "dup Worker out"=w441:refnum<class "TopUI.lvclass">)  [unwired: 7 in]
            n155 = event-data("Discard?"=TRUE) -> ()  [unwired: 1 in, 1 out]
          }
        }
        n156 = call-dynamic "Error Handler.vi"("Worker"=w427, "error_in"=w429) -> ("error out"=w428:errorcluster, "Stop Loop"=w425:bool, "Worker out"=w426:refnum<class "TopUI.lvclass">)  [unwired: 7 in]
      }
    }
    frame Error {
      n157 = call-dynamic "Error Handler.vi"("Worker"=w447, "error_in"=w450) -> ("error out"=w448:errorcluster, "Worker out"=w446:refnum<class "TopUI.lvclass">)  [unwired: 7 in, 1 out]
    }
  }
  n158 = Unregister For Events(event registration refnum=w19, error in=w20) -> (error out=w21:errorcluster)
  n159 = Merge Errors(w21, w14) -> (w18:errorcluster)
  n160 = call-dynamic "Exited Notify and Cleanup.vi"("error_in"=w18, "Worker"=w17) -> ("error out"=→"error out":errorcluster, "dup Worker out"=→"TopUI out":refnum<class "TopUI.lvclass">)  [unwired: 8 in]
